vi "低电量告警对话框.vi"() -> (3 "T button?":bool)   [LabVIEW 2016, in "环境动力监测库.lvlib" / "UPS库.lvlib"]
panel:
  out "告警字符串":string
  in  "取消告警":bool
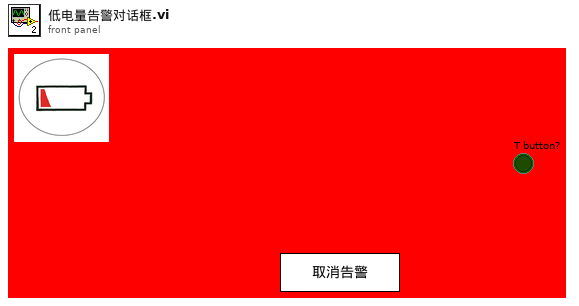
[diagram p1: front panel]
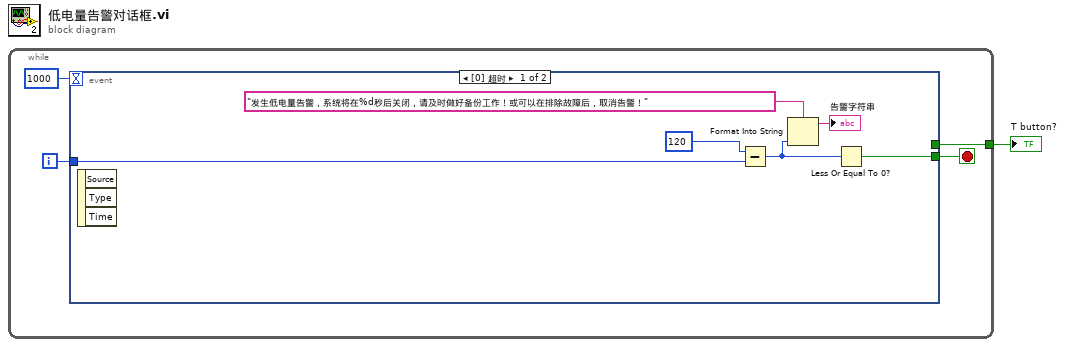
[diagram p0: block diagram]
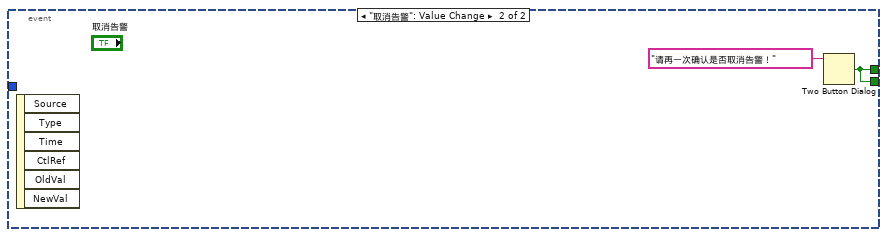
[diagram p2: hidden frame]
diagram:
  n1 = while {
    tunnel: [w5] -> w1
    i -> [w2]
    stop <- w4 stop-if-true
    n2 = event shown="[0] 超时" {
      selector: _ -> [_ _]
      dyn-events: _ -> [_ _]
      timeout: 1000 -> [_ _]
      tunnel: [_ w12] -> w5
      tunnel: [w7 w12] -> w4
      tunnel: w2 -> [w11 _]
      event Timeout {
        n3 = event-data() -> ()  [unwired: 1 in, 3 out]
        n4 = Subtract(x=120, y=w11) -> (x-y=w8:i32)
        n5 = Format Into String(format string="发生低电量告警，系统将在%d秒后关闭，请及时做好备份工作！或可以在排除故障后，取消告警！" ("格式字符串"), w8) -> (resulting string=→"告警字符串":string)  [unwired: 2 in, 1 out]
        n6 = Less Or Equal To 0?(x=w8) -> (x <= 0?=w7:bool)
      }
      event "取消告警": Value Change {
        n7 = event-data() -> ()  [unwired: 1 in, 6 out]
        n8 = Two Button Dialog(message="请再一次确认是否取消告警！" ("消息")) -> (T button?=w12:bool)  [unwired: 2 in]
      }
    }
  }
  "T button?" <- w1
